vi "Unpack Subscription Request.vi"(11 "SubscriptionRequest":refnum<class "SubscriptionRequest.lvclass">) -> (1 "Subscription Policy":T1, 2 "Type":variant, 3 "Datum Name":string)   [LabVIEW 2020, in "MVA Framework.lvlib" / "IMediator.lvlib" / "SubscriptionRequest.lvclass"]
doc: "解除包装订阅请求"
uses:
  SubscriptionRequest.lvclass
  ISubscriptionPolicy/ISubscriptionPolicy Reference.ctl
  ISubscriptionPolicy/ISubscriptionPolicy.lvclass
  SubscriptionRequest.lvclass/SubscriptionRequest.ctl
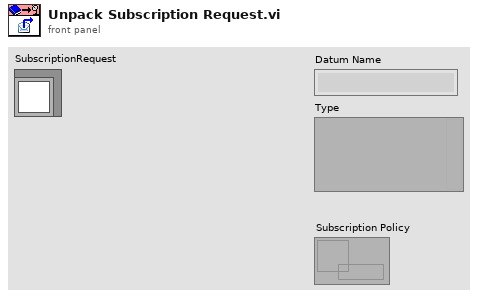
[diagram p1: front panel]
types:
  T1 = typedef "MVA Framework.lvlib/IMediator.lvlib/ISubscriptionPolicy.lvclass/ISubscriptionPolicy Reference.ctl" = refnum<data-value>
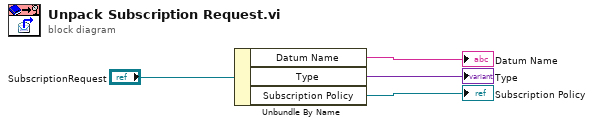
[diagram p0: block diagram]
diagram:
  n1 = Unbundle By Name("SubscriptionRequest") -> ("Datum Name"=→"Datum Name":string, "Type"=→"Type":variant, "Subscription Policy"=→"Subscription Policy":T1)
